vi "OE1022_Configure Auto_Setting.vi"(7 "OE1022_Auto Setting":T1, 8 "Error in (no error)":errorcluster caption="error out（no error）", 9 "Remote Mode":u16(ring) items=["USB"=0, "GPIB"=2], 11 "VISA resource name":refnum<visa-resource-name>) -> (0 "Error out":errorcluster caption="error out", 1 "Output String":string, 3 "VISA resource  out":refnum<visa-resource-name>)   [LabVIEW 2011]
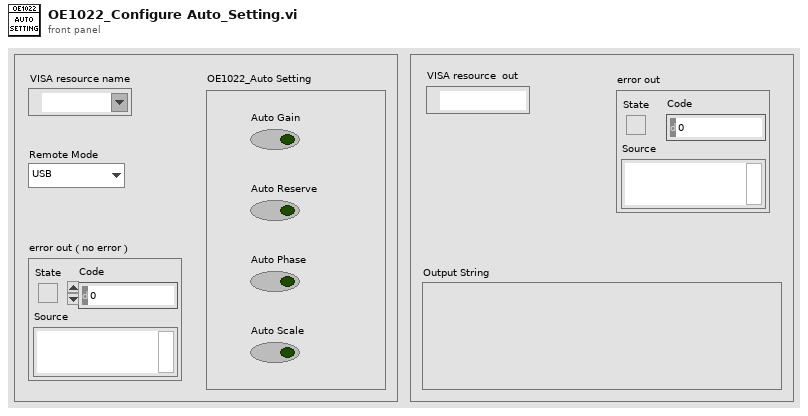
[diagram p1: front panel]
types:
  T1 = cluster{"Auto Gain":bool, "Auto Reserve":bool, "Auto Phase":bool, "Auto Scale":bool}
  T2 = enum16{"ISRC", "IGND", "ICPL", "ILIN", "PHAS", "FMOD", "RSLP", "FREQ", "SWPT", "SLLM", "SULM", "SSLL", "SSLG", "STLM", "SWRM", "IRNG", "SENS", "RMOD", "OFLT", "OFSL", "SYNC", "DMOD", "HARM", "DARB", "SWVT", "SLVL", "SVLL", "SVUL", "SVSL", "SVSG", "SVTM", "SVRM", "RALL", "SNAP", "OUTP", "OAUX", "COUT", "CAUX", "COFP", "CEXP", "FPOP", "OEXP", "*IDN", "*RST", "OVLD", "INOV", "GNOV", "*PLL", "SSET", "RSET", "AGAN", "APHS", "ARSV", "ASCL", "EQCD", "EQCS", "SPED", "SRAT", "SLEN", "SSLE", "STRG", "SPRM", "STRD", "PAUS", "REST", "SPTS", "TRCA", "TEMP", "RSTU", "IHNZ", "DEQU", "SADD", "ARNG", "CSPE", "ISRCD", "IGNDD", "ICPLD", "ILIND", "PHASD", "FMODD", "RSLPD", "FREQD", "SWPTD", "SLLMD", "SULMD", "SSLLD", "SSLGD", "STLMD", "SWRMD", "SENSD", "RMODD", "OFLTD", "OFSLD", "SYNCD", "HARMD", "EQCDD", "EQCSD", "SNAPD", "OUTPD", "SWVTD", "SLVLD", "SVLLD", "SVULD", "SVSLD", "SVSGD", "SVTMD", "SVRMD", "SVDCD", "ARSVD", "AGAND", "APHSD", "ASCLD", "FPOPD", "CAUXD", "OEXPD", "SPEDD", "SRATD", "SLEND", "SSLED", "STRGD", "SPRMD", "STRDD", "PAUSD", "RESTD", "SPTSD", "TRCAD", "*IDND", "*RSTD", "INOVD", "GNOVD", "*PLLD", "SSETD", "RSETD"}
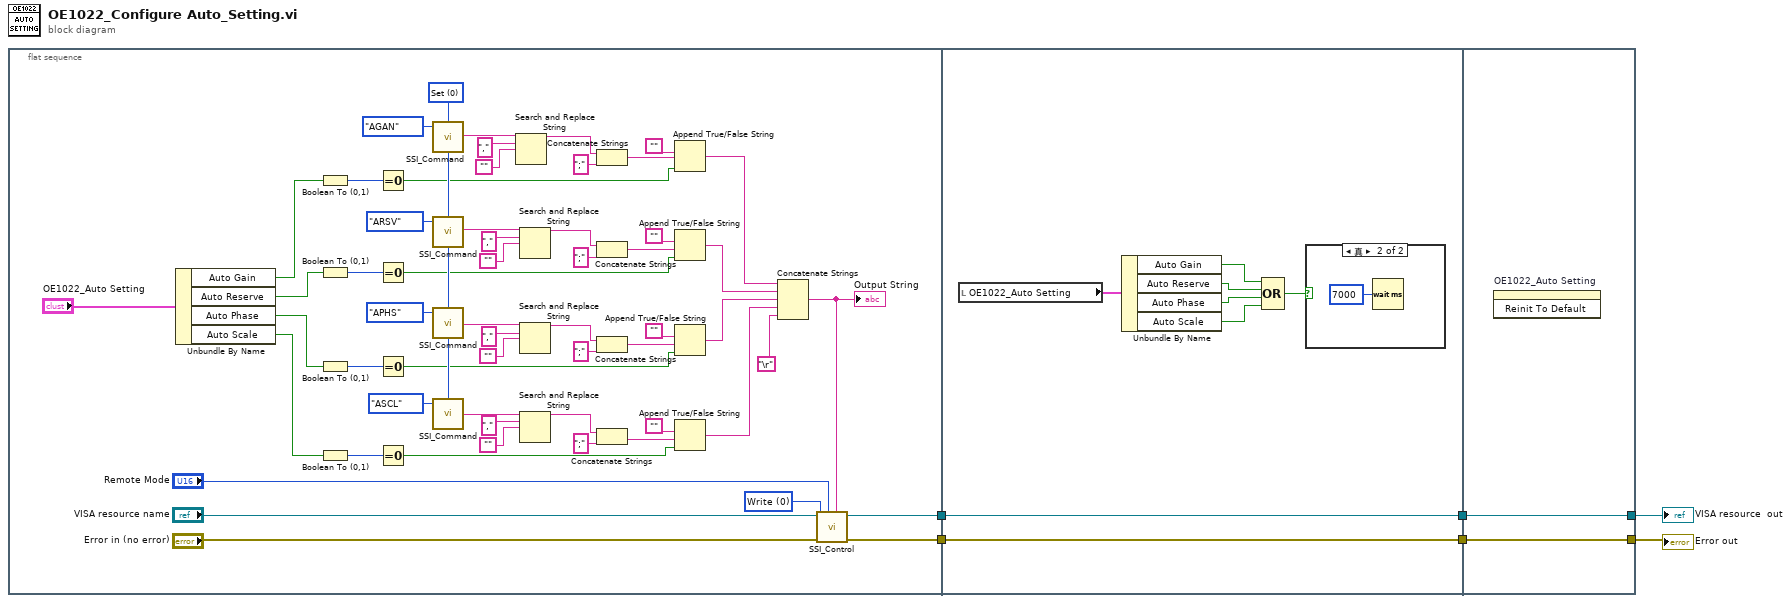
[diagram p0: block diagram]
diagram:
  n1 = flat-sequence {
    tunnel: [w40] -> w6
    tunnel: [w39] -> w5
    tunnel: w6 -> [w72]
    tunnel: w5 -> [w71]
    tunnel: [w72] -> w2
    tunnel: [w71] -> w1
    tunnel: [w74] -> w4
    tunnel: [w75] -> w3
    tunnel: w2 -> [w75]
    tunnel: w1 -> [w74]
    frame #0 {
      w45 = u16 0 items=["Write", "Read"] ("Control")
      w61 = u16 0 items=["Set", "Query"] ("Opera")
      n2 = Unbundle By Name("OE1022_Auto Setting") -> ("Auto Gain"=w63:bool, "Auto Reserve"=w53:bool, "Auto Phase"=w52:bool, "Auto Scale"=w51:bool)
      n3 = Boolean To (0,1)(Boolean=w63) -> (0, 1=w62:i16)
      n4 = Boolean To (0,1)(Boolean=w53) -> (0, 1=w59:i16)
      n5 = Boolean To (0,1)(Boolean=w52) -> (0, 1=w55:i16)
      n6 = Boolean To (0,1)(Boolean=w51) -> (0, 1=w54:i16)
      n7 = Equal To 0?(x=w62) -> (x = 0?=w11:bool)
      n8 = Equal To 0?(x=w59) -> (x = 0?=w12:bool)
      n9 = Equal To 0?(x=w55) -> (x = 0?=w13:bool)
      n10 = Equal To 0?(x=w54) -> (x = 0?=w14:bool)
      n11 = call "SSI_Command.vi"("Opera"=w61, "Command Type"=T2."AGAN") -> ("Output string"=w22:string)  [unwired: 2 in]
      n12 = call "SSI_Command.vi"("Opera"=w61, "Command Type"=T2."ARSV") -> ("Output string"=w15:string)  [unwired: 2 in]
      n13 = call "SSI_Command.vi"("Opera"=w61, "Command Type"=T2."APHS") -> ("Output string"=w17:string)  [unwired: 2 in]
      n14 = call "SSI_Command.vi"("Opera"=w61, "Command Type"=T2."ASCL") -> ("Output string"=w16:string)  [unwired: 2 in]
      n15 = Search and Replace String(input string=w22, search string="," ("搜索字符串"), replace string="") -> (result string=w32:string)  [unwired: 5 in, 3 out]
      n16 = Search and Replace String(input string=w15, search string="," ("搜索字符串"), replace string="") -> (result string=w29:string)  [unwired: 5 in, 3 out]
      n17 = Search and Replace String(input string=w17, search string="," ("搜索字符串"), replace string="") -> (result string=w26:string)  [unwired: 5 in, 3 out]
      n18 = Search and Replace String(input string=w16, search string="," ("搜索字符串"), replace string="") -> (result string=w23:string)  [unwired: 5 in, 3 out]
      n19 = Concatenate Strings(w32, ";") -> (w21:string)
      n20 = Concatenate Strings(w29, ";") -> (w20:string)
      n21 = Concatenate Strings(w26, ";") -> (w19:string)
      n22 = Concatenate Strings(w23, ";") -> (w18:string)
      n23 = Append True/False String(1:w11, 2:w21, 3:"") -> (0:w10:string)  [unwired: 1 in]
      n24 = Append True/False String(1:w12, 2:w20, 3:"") -> (0:w9:string)  [unwired: 1 in]
      n25 = Append True/False String(1:w13, 2:w19, 3:"") -> (0:w8:string)  [unwired: 1 in]
      n26 = Append True/False String(1:w14, 2:w18, 3:"") -> (0:w7:string)  [unwired: 1 in]
      n27 = Concatenate Strings(w10, w9, w8, w7, "\r") -> (w41:string)
      "Output String" <- w41
      n28 = call "SSI_Control.vi"("Write Buffer"=w41, "Remote Mode"="Remote Mode", "Error in (no error)"="Error in (no error)", "Control"=w45, "VISA resource name"="VISA resource name") -> ("Error out"=w39:errorcluster, "VISA resource  out"=w40:refnum<visa-resource-name>)  [unwired: 3 in, 2 out]
    }
    frame #1 {
      n29 = local read "OE1022_Auto Setting"() -> (w70:T1)
      n30 = Unbundle By Name(w70) -> ("Auto Gain"=w68:bool, "Auto Reserve"=w67:bool, "Auto Phase"=w66:bool, "Auto Scale"=w65:bool)
      n31 = Compound Arithmetic op=OR(w68, w67, w66, w65) -> (w69:bool)
      n32 = case shown="真" w69 {
        frame False {
        }
        frame True {
          n33 = Wait (ms)(milliseconds to wait=u32 7000 ("等待时间（毫秒）")) -> ()  [unwired: 1 out]
        }
      }
    }
    frame #2 {
      n34 = invoke on="OE1022_Auto Setting" class="Clust (严格)" method="Reinit To Default"() -> ()  [unwired: 3 in, 3 out]
    }
  }
  "Error out" <- w4
  "VISA resource  out" <- w3
